vi "V7310.Job.Select.vi"(6 "timeout ms (5000)":i32=5000, 8 "error in":errorcluster, 10 "Job":string, 11 "Connection in":refnum<k5>) -> (0 "error out":errorcluster, 1 "VarNames":T1[](array[typedef]), 2 "Jobs":string[](array[string]), 3 "Connection out":refnum<k5>, 5 "Selected Job":string)   [LabVIEW 2016]
uses:
  LowLevel/V7310.Job.Variable.ctl
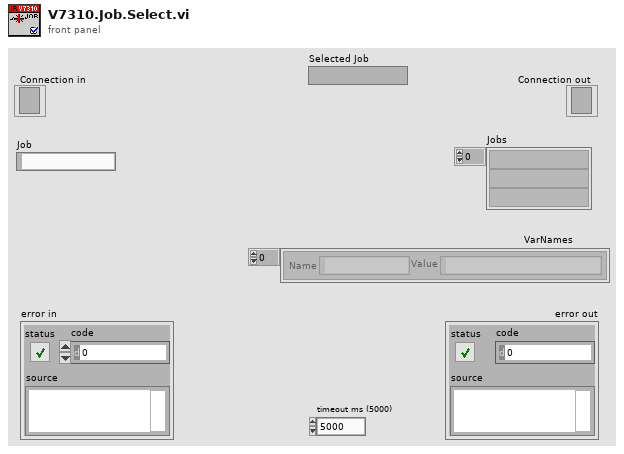
[diagram p1: front panel]
types:
  T1 = typedef "V7310.Job.Variable.ctl" = cluster{"Name":string, "Value":string}
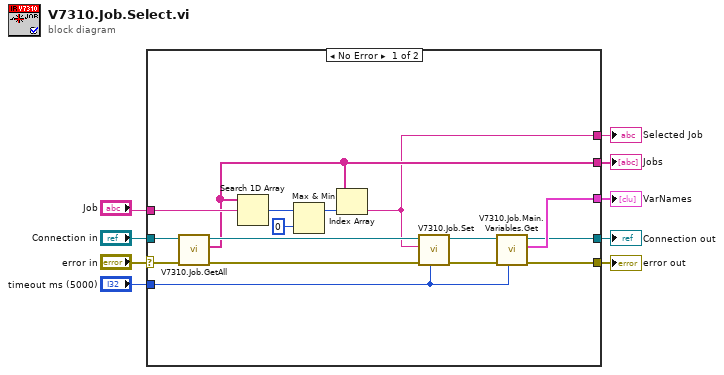
[diagram p0: block diagram]
diagram:
  n1 = case shown="No Error" "error in" {
    selector: "error in" -> [w24 w26]
    tunnel: "Connection in" -> [w23 w27]
    tunnel: [w19 w27] -> w8
    tunnel: "timeout ms (5000)" -> [w18 _]
    tunnel: [w20 w26] -> w5
    tunnel: [w25 _] -> w3
    tunnel: [w12 _] -> w4
    tunnel: "Job" -> [w16 _]
    tunnel: [w10 _] -> w1
    frame No Error {
      n2 = call "V7310.Job.GetAll.vi"("error in"=w24, "Connection in"=w23) -> ("error out"=w17:errorcluster, "Jobs"=w12:string[], "Connection out"=w15:refnum<k5>)  [unwired: 7 in]
      n3 = Search 1D Array(1D array=w12, element=w16) -> (index of element=w14:i32)  [unwired: 1 in]
      n4 = Max & Min(x=w14, y=0) -> (max(x,y)=w11:i32)  [unwired: 1 out]
      n5 = Index Array(array=w12, index=w11) -> (element=w10:string)
      n6 = call "V7310.Job.Set.vi"("timeout ms (5000)"=w18, "error in"=w17, "Job"=w10, "Connection in"=w15) -> ("error out"=w22:errorcluster, "Connection out"=w21:refnum<k5>)  [unwired: 6 in]
      n7 = call "V7310.Job.Main.Variables.Get.vi"("timeout ms (5000)"=w18, "error in"=w22, "Connection in"=w21) -> ("error out"=w20:errorcluster, "VarNames"=w25:T1[], "Connection out"=w19:refnum<k5>)  [unwired: 6 in]
    }
    frame Error {
    }
  }
  "Connection out" <- w8
  "error out" <- w5
  "Jobs" <- w4
  "VarNames" <- w3
  "Selected Job" <- w1
